vi "Exit.vi"(8 "error in (no error)":errorcluster, 11 "Old State":refnum<class "Announcing.lvclass">) -> (0 "error out":errorcluster, 3 "New State":refnum<class "Announcing.lvclass">)   [LabVIEW 2013, in "Receiver.lvlib" / "Receiver Commands Using Processor.lvlib" / "Connect Command.lvlib" / "Announcing.lvclass"]
doc: "This is an abstract method. Override this method to define the behavior when you leave the state."
uses:
  Announcing.lvclass
  Connect Command.lvclass
  Announcing.lvclass/Announcing.ctl
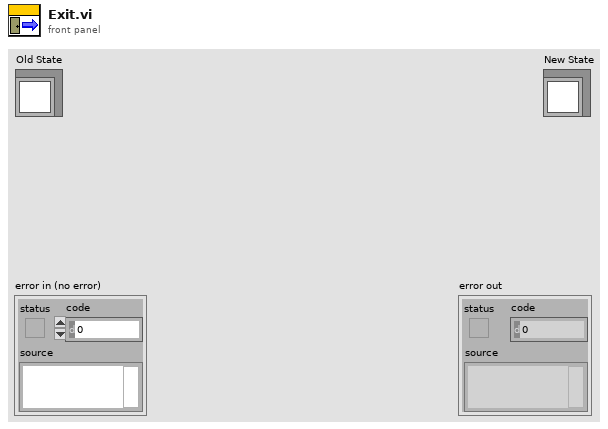
[diagram p1: front panel]
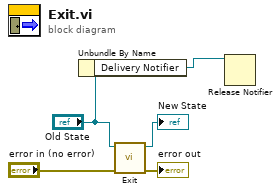
[diagram p0: block diagram]
diagram:
  n1 = Unbundle By Name("Old State") -> ("Delivery Notifier"=w1:refnum<notifier>)
  n2 = call-parent "Exit.vi"("error in (no error)"="error in (no error)", "Old State"="Old State") -> ("error out"=→"error out":errorcluster, "New State"=→"New State":refnum<class "Announcing.lvclass">)  [unwired: 8 in]
  n3 = Release Notifier(notifier=w1) -> ()  [unwired: 2 in, 3 out]
